vi "Write Vpmt.vi"(8 "error in (no error)":errorcluster, 10 "Vpmt":dbl[](array[numeric]), 11 "Change PMT Gain in":refnum<class "Change PMT Gain.lvclass">) -> (0 "error out":errorcluster, 3 "Change PMT Gain out":refnum<class "Change PMT Gain.lvclass">)   [LabVIEW 2014, in "Change PMT Gain.lvclass"]
uses:
  Change PMT Gain.lvclass
  Change PMT Gain.lvclass/Change PMT Gain.ctl
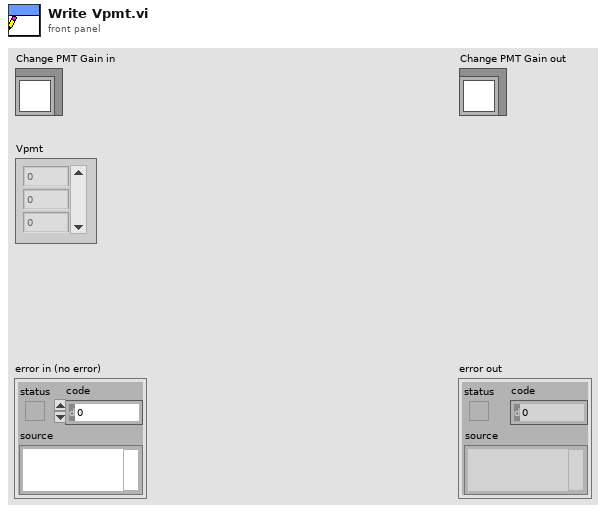
[diagram p1: front panel]
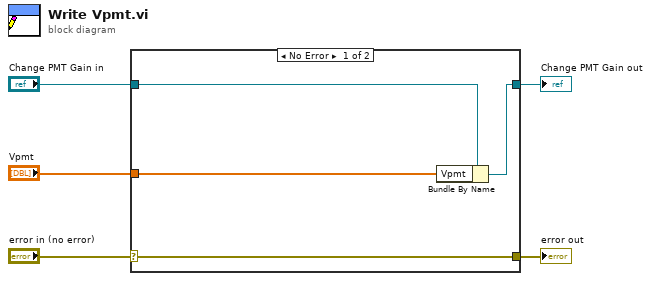
[diagram p0: block diagram]
diagram:
  n1 = case shown="No Error" "error in (no error)" {
    selector: "error in (no error)" -> [w9 w10]
    tunnel: [w9 w10] -> w4
    tunnel: [w7 w11] -> w2
    tunnel: "Change PMT Gain in" -> [w8 w11]
    tunnel: "Vpmt" -> [w6 _]
    frame No Error {
      n2 = Bundle By Name(cluster=w8, "Vpmt"=w6) -> (w7:refnum<class "Change PMT Gain.lvclass">)
    }
    frame Error {
    }
  }
  "error out" <- w4
  "Change PMT Gain out" <- w2
